vi "Write User ID.vi"(8 "Error In":errorcluster) -> (0 "Error Out":errorcluster)   [LabVIEW 2018, in "Tests.lvlib" / "SFTP Attributes.lvlib"]
uses:
  SFTP Attributes.lvlib
  src/Toolkit/SFTP Attributes/SFTP Attributes.lvclass/SFTP Attributes.ctl
  src/Toolkit/SSH/SSH.lvclass/SSH.ctl
  src/Toolkit/SSH/Utility/Read Shared Library.vi
  src/Toolkit/Support/Check Status.vi
  <vilib>/addons/_JKI Toolkits/Caraya/classes/Test/Test.lvclass
  <vilib>/addons/_JKI Toolkits/Caraya/classes/Assert/Assert.lvclass
  src/Toolkit/SFTP Attributes/SFTP Attributes.lvclass
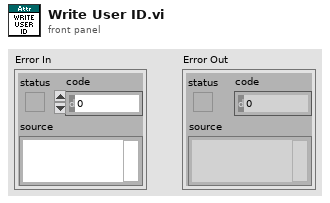
[diagram p1: front panel]
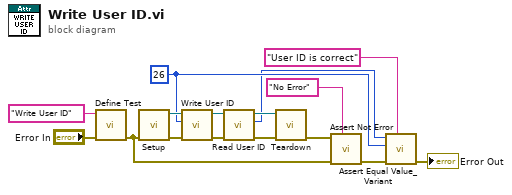
[diagram p0: block diagram]
diagram:
  w2 = u32 26 ("User ID")
  n1 = call <vilib>:"Define Test.vi"("error in (no error)"="Error In", "Label (VI Title)"="Write User ID") -> ("error out"=w12:errorcluster)  [unwired: 9 in]
  n2 = call "Setup.vi"("Error In"=w12) -> ("Error Out"=w8:errorcluster, "SFTP Attributes"=w7:refnum<class "SFTP Attributes.lvclass">)  [unwired: 9 in]
  n3 = call "Write User ID.vi"("Error In"=w8, "User ID"=w2, "SFTP Attributes In"=w7) -> ("Error Out"=w6:errorcluster, "SFTP Attribute Out"=w5:refnum<class "SFTP Attributes.lvclass">)  [unwired: 7 in]
  n4 = call "Read User ID.vi"("Error In"=w6, "SFTP Attributes In"=w5) -> ("Error Out"=w3:errorcluster, "ID"=w1:u32, "SFTP Attribute Out"=w4:refnum<class "SFTP Attributes.lvclass">)  [unwired: 7 in]
  n5 = call "Teardown.vi"("Error In"=w3, "SFTP Attributes"=w4) -> ("Error Out"=w11:errorcluster)  [unwired: 9 in]
  n6 = call <vilib>:"Assert Not Error.vi"("Label"="No Error", "error in (no error)"=w12, "Not Error?"=w11) -> ("error out"=w13:errorcluster)  [unwired: 8 in]
  n7 = call <vilib>:"Assert Equal Value_Variant.vi"("Label"="User ID is correct", "error in (no error)"=w13, "Y"=w2, "X"=w1) -> ("error out"=→"Error Out":errorcluster)  [unwired: 7 in]
